vi "DK240 GratingSelect.vi"(4 "error in":errorcluster, 5 "RésAct":T1(ring)=enum."Réseaux 3" caption="Réseaux désiré", 6 "MovingRef":refnum<vi>, 7 "Port":refnum<visa-resource-name>="SPECTRO") -> (0 "error out":errorcluster, 2 "Moving":bool caption="Déplacement\nen cours", 3 "Status":u8)   [LabVIEW 2019]
doc: "Ce VI permet la sélection du réseaux."
uses:
  <vilib>/Utility/error.llb/DialogType.ctl
panel:
  out "Cancel":u8
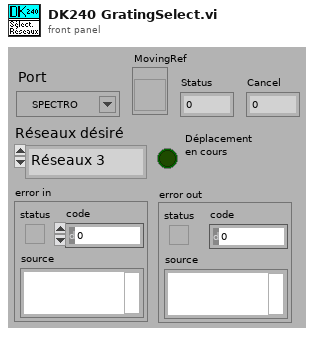
[diagram p1: front panel]
types:
  T1 = enum16{"Réseaux 1", "Réseaux 2", "Réseaux 3", "Échec"}
  T2 = enum16{"Commande", "AttendPrêt", "Paramètre", "AttendFin", "Statut", "Fin"}
  T3 = typedef "DialogType.ctl" = u16
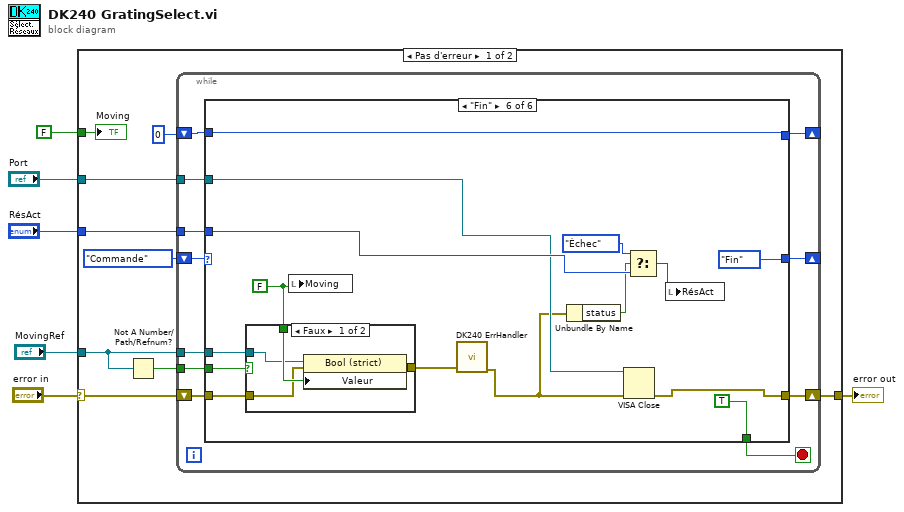
[diagram p0: block diagram]
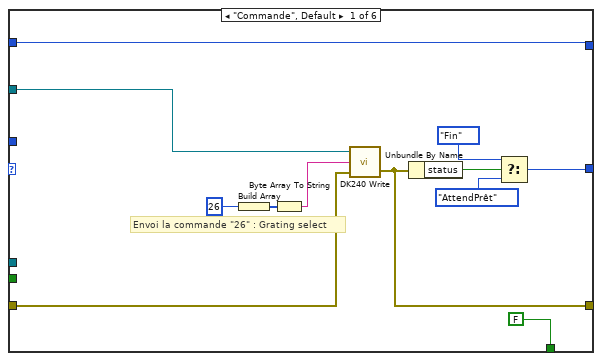
[diagram p2: hidden frame]
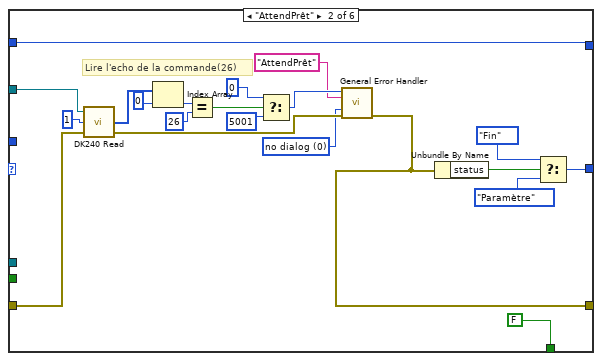
[diagram p3: hidden frame]
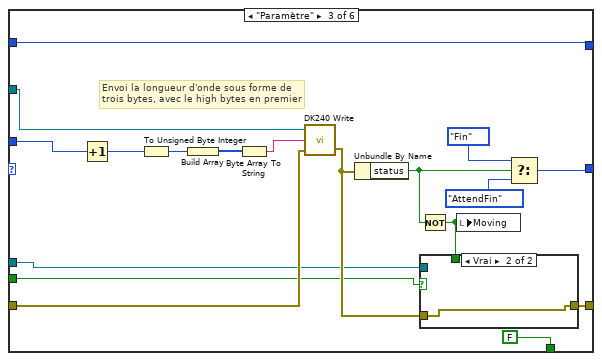
[diagram p4: hidden frame]
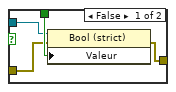
[diagram p5: hidden frame]
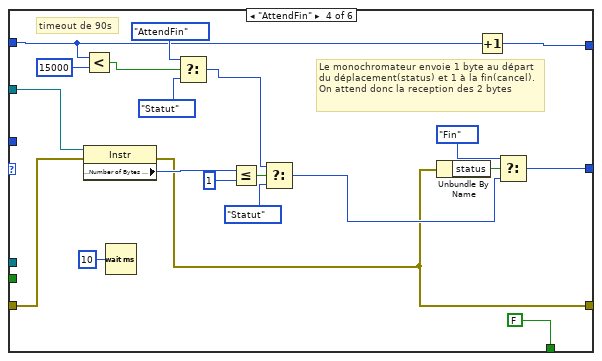
[diagram p6: hidden frame]
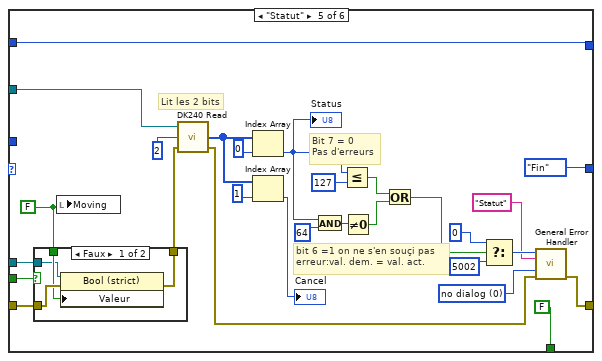
[diagram p7: hidden frame]
diagram:
  n1 = case shown="Pas d'erreur" "error in" {
    selector: "error in" -> [w12 w156]
    tunnel: "Port" -> [w14 _]
    tunnel: [w13 w156] -> w5
    tunnel: FALSE ("Moving") -> [w11 _]
    tunnel: "RésAct" -> [w10 _]
    tunnel: "MovingRef" -> [w9 _]
    frame No Error {
      n2 = Not A Number/Path/Refnum?(number/path/refnum=w9) -> (NaN/Path/Refnum?=w8:bool)
      n3 = while {
        shift-right: [w22] -> _
        shift-left: T2."Commande" -> [w26]
        tunnel: w14 -> [w25]
        shift-right: [w23] -> w13
        shift-left: w12 -> [w24]
        tunnel: w10 -> [w20]
        tunnel: w9 -> [w19]
        tunnel: w8 -> [w18]
        shift-right: [w16] -> _
        shift-left: 0 -> [w17]
        stop <- w21 stop-if-true
        n4 = case shown="\"Fin\"" w26 {
          tunnel: w25 -> [w35 w52 w75 w94 w126 w142]
          tunnel: w24 -> [w34 w51 w74 w102 w108 w147]
          tunnel: [w33 w47 w67 w91 w115 w143] -> w23
          tunnel: [w29 w56 w71 w95 T2."Fin" T2."Fin"] -> w22
          tunnel: [FALSE FALSE FALSE FALSE FALSE TRUE] -> w21
          tunnel: w20 -> [_ _ w65 _ _ w146]
          tunnel: w19 -> [_ _ w61 _ w104 w140]
          tunnel: w18 -> [_ _ w60 _ w105 w141]
          tunnel: w17 -> [w27 w39 w62 w87 w103 w139]
          tunnel: [w27 w39 w62 w88 w103 w139] -> w16
          frame "Commande", Default {
            # "Envoi la commande \"26\" : Grating select"
            n5 = Build Array(u8 26) -> (w37:u8[])
            n6 = Byte Array To String(unsigned byte array=w37) -> (string=w38:string)
            n7 = call <userlib>:"DK240 Write.vi"("error in"=w34, "String to write"=w38, "Port"=w35) -> ("error out"=w33:errorcluster)  [unwired: 1 in]
            n8 = Unbundle By Name(w33) -> ("status"=w32:bool)
            n9 = Select(t=T2."Fin", s=w32, f=T2."AttendPrêt") -> (s? t:f=w29:T2)
          }
          frame "AttendPrêt" {
            w41 = T3 0 items=["no dialog", "OK message", "continue or stop message", "OK message + warnings", "continue/stop + warnings"] ("type of dialog (OK msg:1)")
            # "Lire l'echo de la commande(26)"
            n10 = call <userlib>:"DK240 Read.vi"("error in"=w51, "Byte count"=u32 1, "Port"=w52) -> ("error out"=w48:errorcluster, "Received Bytes"=w55:u8[])  [unwired: 1 in]
            n11 = Index Array(array=w55, index=0) -> (element=w50:u8)
            n12 = Equal?(x=w50, y=u8 26) -> (x = y?=w46:bool)
            n13 = Select(t=0, s=w46, f=5001 ("t")) -> (s? t:f=w45:i32)
            n14 = call <vilib>:"General Error Handler.vi"("[error code] (0)"=w45, "[error source] (\" \")"="AttendPrêt" ("[error source] (\" \")"), "type of dialog (OK msg:1)"=w41, "error in (no error)"=w48) -> ("error out"=w47:errorcluster)  [unwired: 7 in, 4 out]
            n15 = Unbundle By Name(w47) -> ("status"=w59:bool)
            n16 = Select(t=T2."Fin", s=w59, f=T2."Paramètre") -> (s? t:f=w56:T2)
          }
          frame "Paramètre" {
            # "Envoi la longueur d'onde sous forme de trois bytes, avec le high bytes en premier"
            n17 = Increment(x=w65) -> (x+1=w63:T1)
            n18 = To Unsigned Byte Integer(number=w63) -> (unsigned 8bit integer=w64:u8)
            n19 = Build Array(w64) -> (w76:u8[])
            n20 = Byte Array To String(unsigned byte array=w76) -> (string=w77:string)
            n21 = call <userlib>:"DK240 Write.vi"("error in"=w74, "String to write"=w77, "Port"=w75) -> ("error out"=w66:errorcluster)  [unwired: 1 in]
            n22 = Unbundle By Name(w66) -> ("status"=w69:bool)
            n23 = Not(x=w69) -> (.not. x?=w68:bool)
            n24 = case shown="Vrai" w60 {
              tunnel: w68 -> [w81 _]
              tunnel: [w80 w82] -> w67
              tunnel: w66 -> [w79 w82]
              tunnel: w61 -> [w78 _]
              frame False {
                n25 = property class="Bool (strict)"(reference=w78, error in=w79, "Valeur"=w81) -> (error out=w80:errorcluster)  [unwired: 1 out]
              }
              frame True {
              }
            }
            n26 = local write "Moving"(w68) -> ()
            n27 = Select(t=T2."Fin", s=w69, f=T2."AttendFin") -> (s? t:f=w71:T2)
          }
          frame "AttendFin" {
            # "timeout de 90s"
            # "Le monochromateur envoie 1 byte au départ du déplacement(status) et 1 à la fin(cancel). On attend donc la reception des 2 bytes"
            n28 = Less?(x=w87, y=15000) -> (x < y?=w85:bool)
            n29 = property class="Instr"(reference=w94, error in=w102) -> (error out=w91:errorcluster, "Serial Settings:Number of Bytes at Serial Port"=w101:u32)  [unwired: 1 out]
            n30 = Wait (ms)(milliseconds to wait=u32 10) -> ()  [unwired: 1 out]
            n31 = Select(t=T2."AttendFin", s=w85, f=T2."Statut") -> (s? t:f=w84:T2)
            n32 = Less Or Equal?(x=w101, y=u32 1) -> (x <= y?=w97:bool)
            n33 = Select(t=w84, s=w97, f=T2."Statut") -> (s? t:f=w92:T2)
            n34 = Unbundle By Name(w91) -> ("status"=w99:bool)
            n35 = Increment(x=w87) -> (x+1=w88:i32)
            n36 = Select(t=T2."Fin", s=w99, f=w92) -> (s? t:f=w95:T2)
          }
          frame "Statut" {
            w120 = T3 0 items=["no dialog", "OK message", "continue or stop message", "OK message + warnings", "continue/stop + warnings"] ("type of dialog (OK msg:1)")
            w107 = FALSE
            # "bit 6 =1 on ne s'en souçi pas \nerreur:val. dem. = val. act."
            # "Bit 7 = 0\nPas d'erreurs"
            # "Lit les 2 bits"
            n37 = case shown="Faux" w105 {
              tunnel: w108 -> [w134 w135]
              tunnel: w107 -> [w133 _]
              tunnel: [w132 w135] -> w106
              tunnel: w104 -> [w131 _]
              frame False {
                n38 = property class="Bool (strict)"(reference=w131, error in=w134, "Valeur"=w133) -> (error out=w132:errorcluster)  [unwired: 1 out]
              }
              frame True {
              }
            }
            n39 = local write "Moving"(w107) -> ()
            n40 = call <userlib>:"DK240 Read.vi"("error in"=w106, "Byte count"=u32 2, "Port"=w126) -> ("error out"=w119:errorcluster, "Received Bytes"=w130:u8[])  [unwired: 1 in]
            n41 = Index Array(array=w130, index=0) -> (element=w111:u8)
            "Status" <- w111
            n42 = Index Array(array=w130, index=1) -> (element=→"Cancel":u8)
            n43 = And(x=w111, y=u8 64) -> (x .and. y?=w117:u8)
            n44 = Less Or Equal?(x=w111, y=u8 127) -> (x <= y?=w114:bool)
            n45 = Not Equal To 0?(x=w117) -> (x != 0?=w113:bool)
            n46 = Or(x=w114, y=w113) -> (x .or. y?=w112:bool)
            n47 = Select(t=0, s=w112, f=5002 ("t")) -> (s? t:f=w124:i32)
            n48 = call <vilib>:"General Error Handler.vi"("[error code] (0)"=w124, "[error source] (\" \")"="Statut" ("[error source] (\" \")"), "type of dialog (OK msg:1)"=w120, "error in (no error)"=w119) -> ("error out"=w115:errorcluster)  [unwired: 7 in, 4 out]
          }
          frame "Fin" {
            w148 = FALSE
            n49 = case shown="Faux" w141 {
              tunnel: w148 -> [w154 _]
              tunnel: w147 -> [w153 w155]
              tunnel: [w152 w155] -> w138
              tunnel: w140 -> [w151 _]
              frame False {
                n50 = property class="Bool (strict)"(reference=w151, error in=w153, "Valeur"=w154) -> (error out=w152:errorcluster)  [unwired: 1 out]
              }
              frame True {
              }
            }
            n51 = local write "Moving"(w148) -> ()
            n52 = call <userlib>:"DK240 ErrHandler.vi"("error in"=w138) -> ("error out"=w137:errorcluster)  [unwired: 7 in]
            n53 = Unbundle By Name(w137) -> ("status"=w136:bool)
            n54 = VISA Close(VISA resource name=w142, error in (no error)=w137) -> (error out=w143:errorcluster)
            n55 = Select(t=T1."Échec", s=w136, f=w146) -> (s? t:f=w145:T1)
            n56 = local write "RésAct"(w145) -> ()
          }
        }
      }
      "Moving" <- w11
    }
    frame Error {
    }
  }
  "error out" <- w5
